vi "Write NPin 1Samp 1D Boolean.vi"(8 "error in (no error)":errorcluster, 9 "values":bool[](array[boolean]), 10 "Pins":u8[](array[numeric]), 11 "MicroDAQ.lvlib:Digital output.lvclass":refnum<class "Digital output.lvclass">) -> (0 "error out":errorcluster, 3 "MicroDAQ.lvlib:Digital output.lvclass out":refnum<class "Digital output.lvclass">)   [LabVIEW 2009, in "MicroDAQ.lvlib" / "Digital output.lvclass"]
doc: "Writes a array of Boolean samples to a digital output channel composed of a multiple lines."
uses:
  <instrlib>/MicroDAQ/Channel/Digital output/Digital output.lvclass
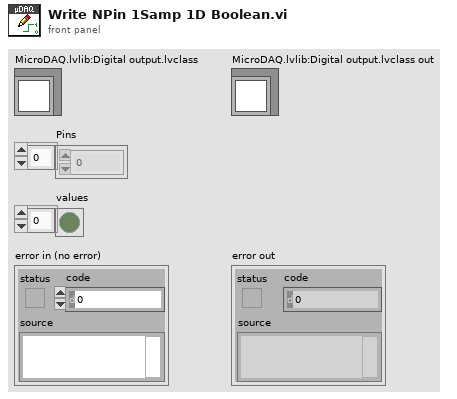
[diagram p1: front panel]
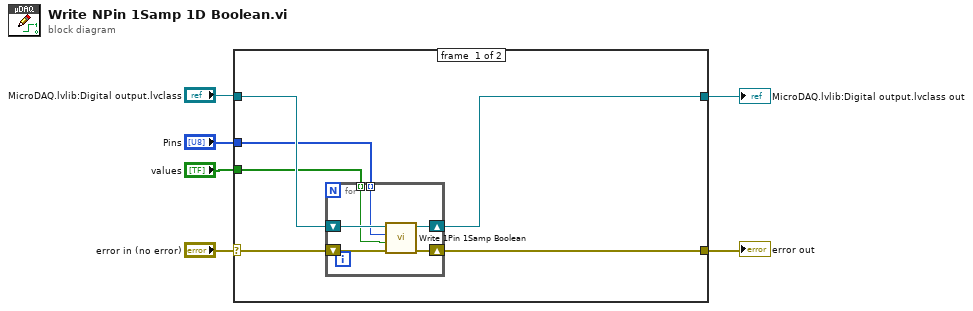
[diagram p0: block diagram]
diagram:
  n1 = case shown="No Error" "error in (no error)" {
    selector: "error in (no error)" -> [w12 w19]
    tunnel: [w11 w19] -> w5
    tunnel: "MicroDAQ.lvlib:Digital output.lvclass" -> [w9 w20]
    tunnel: [w10 w20] -> w3
    tunnel: "Pins" -> [w8 _]
    tunnel: "values" -> [w7 _]
    frame #0 {
      n2 = for {
        shift-right: [w17] -> w11
        shift-left: w12 -> [w18]
        shift-right: [w16] -> w10
        shift-left: w9 -> [w15]
        tunnel: w8 -> [w14] mode=indexing
        tunnel: w7 -> [w13] mode=indexing
        n3 = call <instrlib>:"Write 1Pin 1Samp Boolean.vi"("error in (no error)"=w18, "data"=w13, "Pin"=w14, "MicroDAQ.lvlib:Digital output.lvclass"=w15) -> ("error out"=w17:errorcluster, "MicroDAQ.lvlib:Digital output.lvclass out"=w16:refnum<class "Digital output.lvclass">)  [unwired: 6 in]
      }
    }
    frame #1 {
    }
  }
  "error out" <- w5
  "MicroDAQ.lvlib:Digital output.lvclass out" <- w3
